vi "WFComposeA.vi"(8 "error in (no error)":errorcluster, 9 "WFRepetitions":T2={"Del (s)"=0.0, "Int (s)"=0.0, "N"=1} {"Int (s)" min=0.0 format="%#_4g"; "Del (s)" min=0.0 format="%#_4f"}, 10 "WFParameters":T1={"Fs (Hz)"=100000.0, "Amp (V)"=1.0, "Ramp (s)"=0.005, "Dur (s)"=0.25, "Baseline (V)"=0.0} {"Dur (s)" min=0.0 format="%#_4g"; "Ramp (s)" min=0.0; "Fs (Hz)" min=0.0}, 11 "Waveform In":waveform(dbl)={"t0"=timestamp(0 s since 1904-01-01), "dt"=0.0, "Y"=[]}) -> (0 "error out":errorcluster, 3 "Analog Waveform Out":waveform(dbl))   [LabVIEW 2013]
uses:
  WFRepetitions.ctl
  WFParameters.ctl
  WFComposeCanA.vi
  WFAppend2A.vi
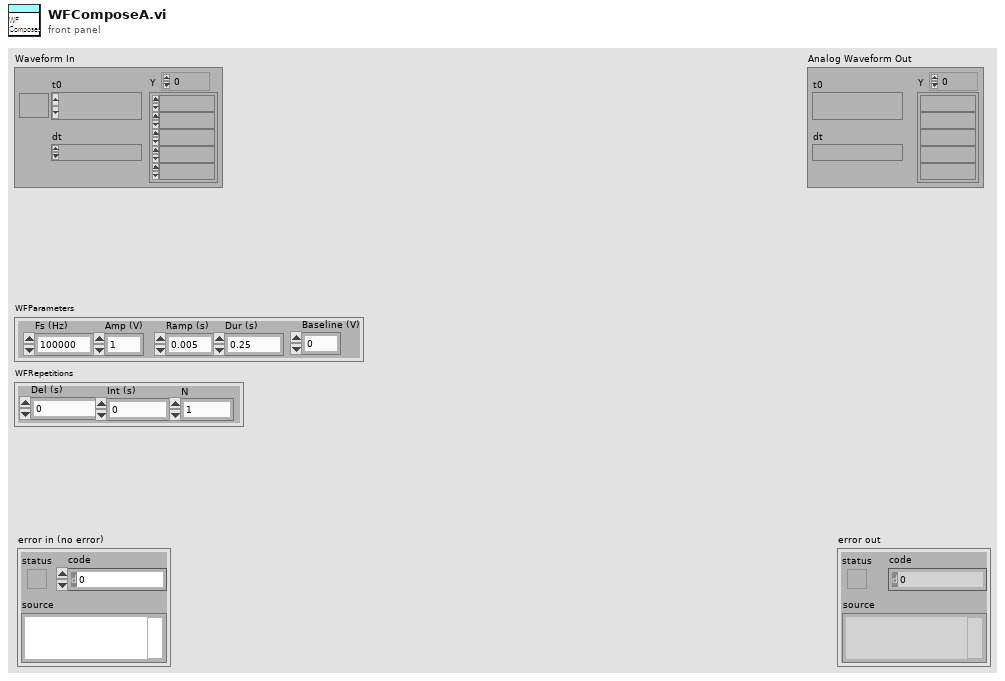
[diagram p1: front panel]
types:
  T1 = typedef "WFParameters.ctl" = cluster{"Fs (Hz)":dbl, "Amp (V)":dbl, "Ramp (s)":dbl, "Dur (s)":dbl, "Baseline (V)":dbl}
  T2 = typedef "WFRepetitions.ctl" = cluster{"Del (s)":dbl, "Int (s)":dbl, "N":i32}
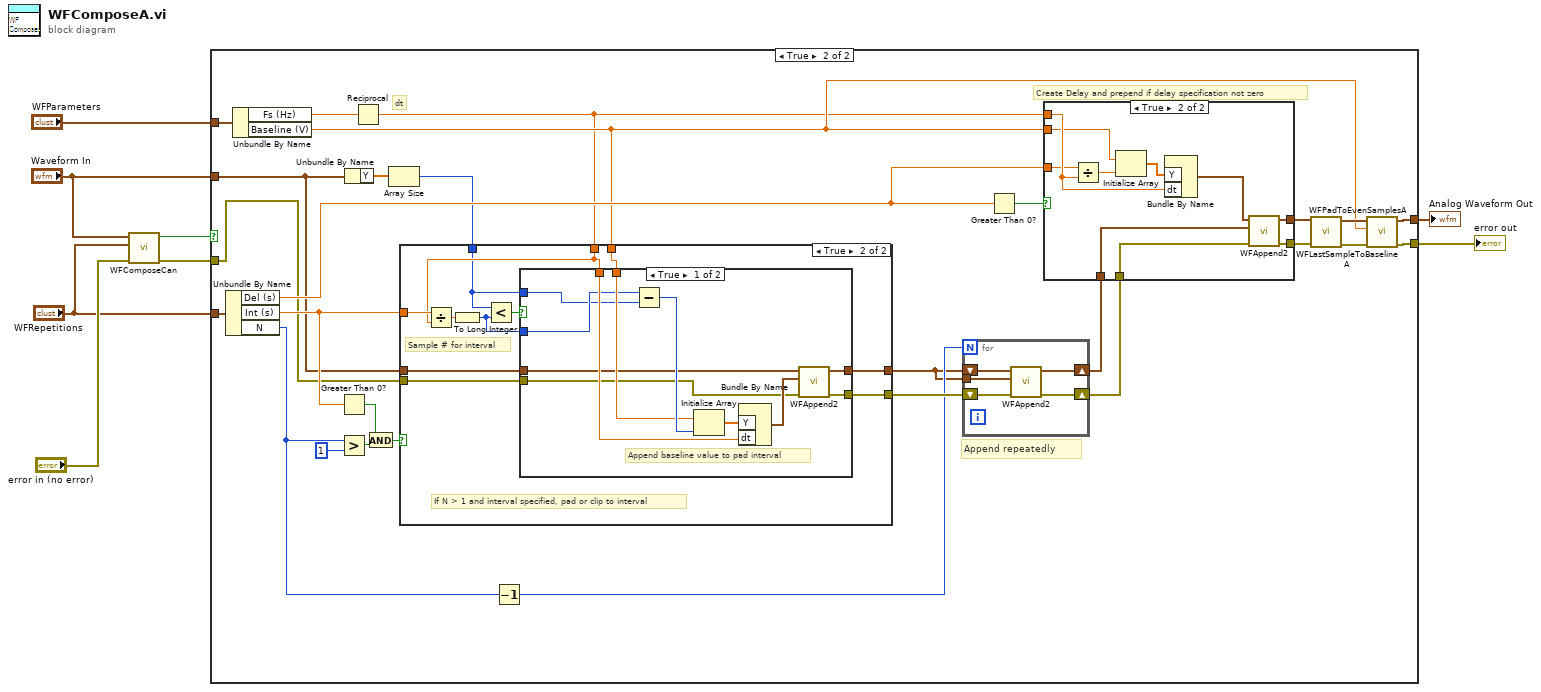
[diagram p0: block diagram]
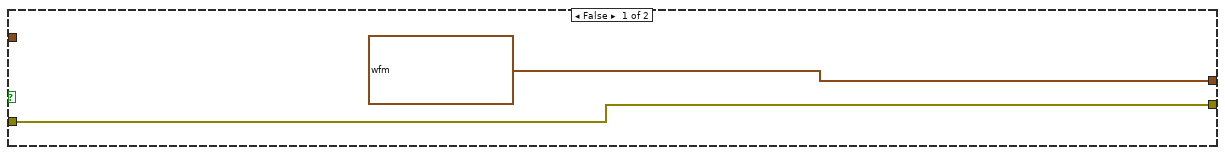
[diagram p2: hidden frame]
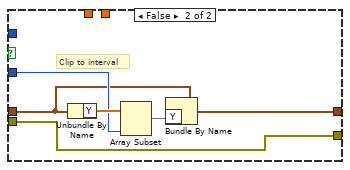
[diagram p4: hidden frame]
diagram:
  n1 = call-poly "WFComposeCan.vi"("error in (no error)"="error in (no error)", "WFRepetitions"="WFRepetitions", "Waveform In"="Waveform In") -> ("error out"=w5:errorcluster, "ComposeCan"=w7:bool)  [unwired: 7 in]
  n2 = case shown="True" w7 {
    tunnel: [waveform(dbl) {"t0"=timestamp(0 s since 1904-01-01), "dt"=1.0, "Y"=[]} ("Waveform") w26] -> w8
    tunnel: w5 -> [w9 w13]
    tunnel: [w9 w27] -> w4
    tunnel: "Waveform In" -> [_ w14]
    tunnel: "WFRepetitions" -> [_ w36]
    tunnel: "WFParameters" -> [_ w24]
    frame False {
    }
    frame True {
      # "dt"
      # "Append repeatedly"
      # "Create Delay and prepend if delay specification not zero"
      n3 = Unbundle By Name(w36) -> ("Del (s)"=w31:dbl, "Int (s)"=w15:dbl, "N"=w19:i32)
      n4 = Unbundle By Name(w24) -> ("Fs (Hz)"=w23:dbl, "Baseline (V)"=w22:dbl)
      n5 = Greater Than 0?(x=w15) -> (x > 0?=w16:bool)
      n6 = Greater?(x=w19, y=1) -> (0:w17:bool)
      n7 = Unbundle By Name(w14) -> ("Y"=w12:dbl[])
      n8 = Reciprocal(x=w23) -> (1/x=w21:dbl)
      n9 = And(x=w16, y=w17) -> (x .and. y?=w20:bool)
      n10 = Array Size(array=w12) -> (size(s)=w11:i32)
      n11 = case shown="True" w20 {
        tunnel: [w39 w51] -> w37
        tunnel: [w40 w49] -> w34
        tunnel: w22 -> [_ w48]
        tunnel: w15 -> [_ w47]
        tunnel: w21 -> [_ w46]
        tunnel: w11 -> [_ w44]
        tunnel: w14 -> [w40 w42]
        tunnel: w13 -> [w39 w41]
        frame False {
          # "If N = 1 or interval not specified, just pass through"
        }
        frame True {
          # "If N > 1 and interval specified, pad or clip to interval"
          # "Sample # for interval"
          n12 = Divide(x=w47, y=w46) -> (x/y=w45:dbl)
          n13 = To Long Integer(number=w45) -> (32bit integer=w43:i32)
          n14 = Less?(x=w44, y=w43) -> (x < y?=w50:bool)
          n15 = case shown="True" w50 {
            tunnel: w46 -> [w61 _]
            tunnel: [w58 w63] -> w51
            tunnel: [w57 w66] -> w49
            tunnel: w48 -> [w56 _]
            tunnel: w44 -> [w52 _]
            tunnel: w43 -> [w53 w67]
            tunnel: w42 -> [w55 w65]
            tunnel: w41 -> [w54 w63]
            frame True {
              # "Append baseline value to pad interval"
              n16 = Subtract(x=w53, y=w52) -> (x-y=w60:i32)
              n17 = Initialize Array(w56, w60) -> (w62:dbl[])
              n18 = Bundle By Name("Y"=w62, "dt"=w61) -> (w59:waveform(dbl))  [unwired: 1 in]
              n19 = call-poly "WFAppend2.vi"("error in (no error)"=w54, "Waveform In 2"=w59, "Waveform In"=w55) -> ("error out"=w58:errorcluster, "Waveform Out"=w57:waveform(dbl))  [unwired: 3 in]
            }
            frame False {
              # "Clip to interval"
              n20 = Unbundle By Name(w65) -> ("Y"=w68:dbl[])
              n21 = Array Subset(array=w68, length=w67) -> (w64:dbl[])  [unwired: 1 in]
              n22 = Bundle By Name(cluster=w65, "Y"=w64) -> (w66:waveform(dbl))
            }
          }
        }
      }
      n23 = Decrement(x=w19) -> (x-1=w35:i32)
      n24 = for {
        N: w35 -> [_]
        shift-right: [w72] -> w33
        shift-left: w34 -> [w73]
        shift-right: [w70] -> w32
        shift-left: w37 -> [w71]
        tunnel: w34 -> [w69]
        n25 = call-poly "WFAppend2.vi"("error in (no error)"=w71, "Waveform In 2"=w69, "Waveform In"=w73) -> ("error out"=w70:errorcluster, "Waveform Out"=w72:waveform(dbl))  [unwired: 3 in]
      }
      n26 = Greater Than 0?(x=w31) -> (x > 0?=w38:bool)
      n27 = case shown="True" w38 {
        tunnel: w21 -> [_ w83]
        tunnel: w33 -> [w75 w81]
        tunnel: [w75 w80] -> w30
        tunnel: w32 -> [w74 w79]
        tunnel: [w74 w78] -> w29
        tunnel: w31 -> [_ w77]
        tunnel: w22 -> [_ w76]
        frame False {
        }
        frame True {
          n28 = Divide(x=w77, y=w83) -> (x/y=w84:dbl)
          n29 = Initialize Array(w76, w84) -> (w85:dbl[])
          n30 = Bundle By Name("Y"=w85, "dt"=w83) -> (w82:waveform(dbl))  [unwired: 1 in]
          n31 = call-poly "WFAppend2.vi"("error in (no error)"=w79, "Waveform In 2"=w81, "Waveform In"=w82) -> ("error out"=w78:errorcluster, "Waveform Out"=w80:waveform(dbl))  [unwired: 3 in]
        }
      }
      n32 = call "WFPadToEvenSamplesA.vi"("error in (no error)"=w29, "Waveform In"=w30) -> ("error out"=w28:errorcluster, "Waveform Out"=w25:waveform(dbl))  [unwired: 4 in]
      n33 = call "WFLastSampleToBaselineA.vi"("error in (no error)"=w28, "Baseline"=w22, "Waveform In"=w25) -> ("error out"=w27:errorcluster, "Waveform Out"=w26:waveform(dbl))  [unwired: 3 in]
    }
  }
  "error out" <- w4
  "Analog Waveform Out" <- w8
